vi "SwitchAlias.vi"(0 "reference in":refnum<class "SwitchBase.lvclass">, 1 "Name":string, 2 "Connect":bool, 5 "error in (no error)":errorcluster) -> (14 "reference in":refnum<class "SwitchBase.lvclass">, 19 "error out":errorcluster)   [LabVIEW 2017]
uses:
  SwitchBase.lvclass
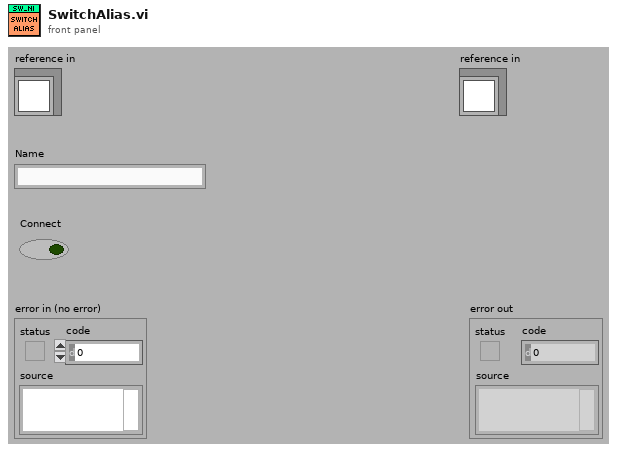
[diagram p1: front panel]
types:
  T1 = typedef "SwitchBase.lvlib/SwitchBase.lvclass/ObjectAttributes.ctl" = cluster{"Config":T2, "History":string[], "channel 1":string, "channel 2":string, "ActiveAlias":string, "AliasState":bool}
  T2 = typedef "SwitchBase.lvlib/SwitchBase.lvclass/Config.ctl" = cluster{"Resource":refnum<k15>, "topology name":T3, "Alias":cluster{"Name":string, "C1,C2":string[][]}[]}
  T3 = typedef "niSwitch Topologies.ctl" = string
  T4 = typedef "SwitchBase.lvlib/SwitchBase.lvclass/ObjectAttributes.ctl" = cluster{"Numeric":dbl}
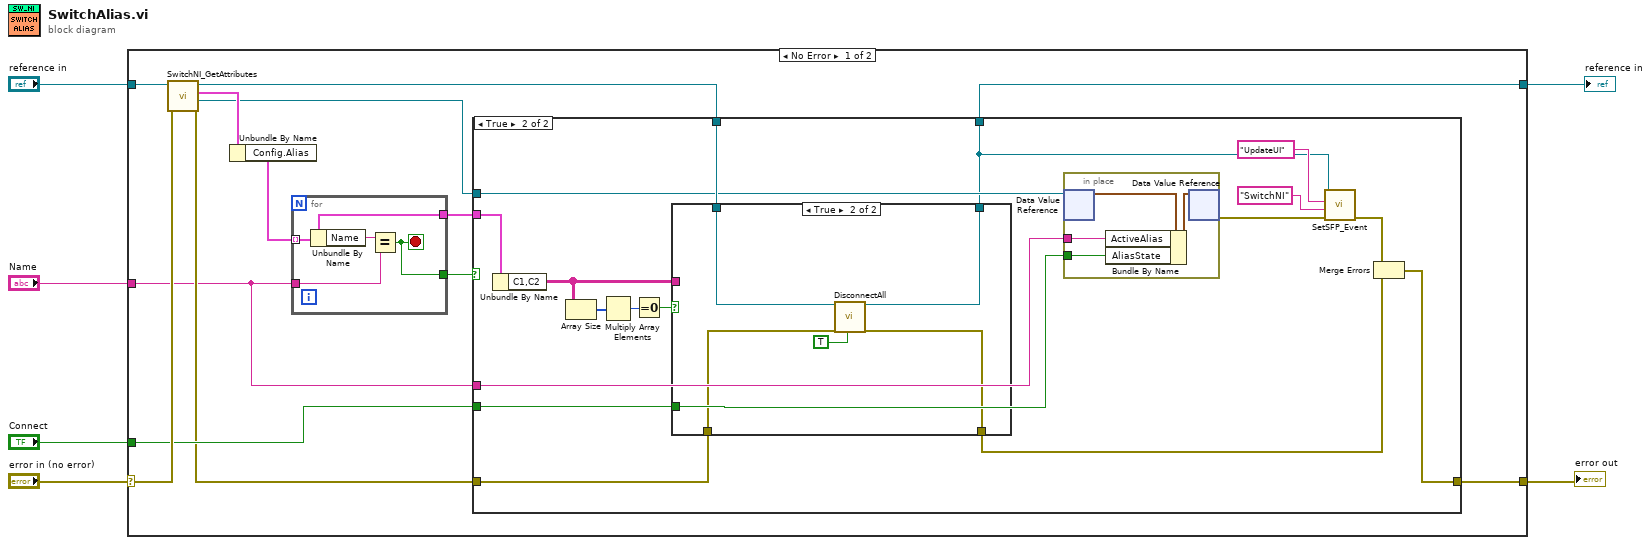
[diagram p0: block diagram]
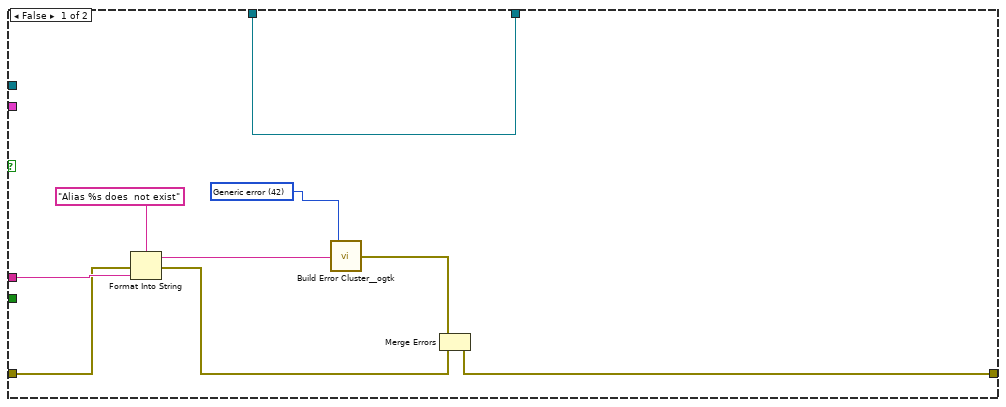
[diagram p2: hidden frame]
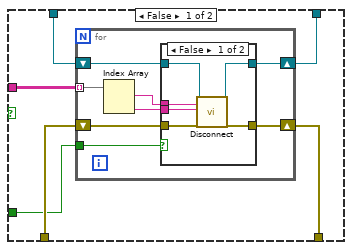
[diagram p3: hidden frame]
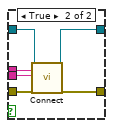
[diagram p4: hidden frame]
diagram:
  n1 = case shown="No Error" "error in (no error)" {
    selector: "error in (no error)" -> [w19 w86]
    tunnel: [w9 w86] -> w5
    tunnel: [w11 w85] -> w3
    tunnel: "reference in" -> [w17 w85]
    tunnel: "Name" -> [w8 _]
    tunnel: "Connect" -> [w13 _]
    frame No Error {
      n2 = call "SwitchNI_GetAttributes.vi"("error in (no error)"=w19, "reference in"=w17) -> ("error out"=w10:errorcluster, "DataRef"=w7:refnum<data-value>, "Data"=w18:T1, "reference out"=w12:refnum<class "SwitchBase.lvclass">)  [unwired: 6 in]
      n3 = Unbundle By Name(w18) -> ("Config.Alias"=w16:cluster{"Name":string, "C1,C2":string[][]}[])
      n4 = for {
        tunnel: w16 -> [w82] mode=indexing
        tunnel: w8 -> [w83]
        tunnel: [w82] -> w14
        tunnel: [w81] -> w15
        stop <- w81 stop-if-true
        n5 = Unbundle By Name(w82) -> ("Name"=w84:string)
        n6 = Equal?(x=w84, y=w83) -> (x = y?=w81:bool)
      }
      n7 = case shown="True" w15 {
        tunnel: w14 -> [_ w43]
        tunnel: w13 -> [_ w40]
        tunnel: w12 -> [w28 w45]
        tunnel: [w28 w29] -> w11
        tunnel: w10 -> [w23 w44]
        tunnel: [w26 w30] -> w9
        tunnel: w8 -> [w24 w41]
        tunnel: w7 -> [_ w42]
        frame False {
          w25 = 42 items=["No error", "Argument error", "Memory is full", "Out of zone", "End of file", "File already open", "Generic file I/O error", "File not found", "File permission error", "Disk is full", "Duplicate path", "Too many files open", "System feature not enabled", "Resource file not found", "Cannot add resource", "Resource not found", "Image not found", "Image memory error", "Pen does not exist", "Config type invalid", "Config token not found", "Config parse error", "Config memory error", "Bad external code format", "Bad external code offset", "External code not present", "Null window", "Destroy window error", "Null menu", "Print aborted", "Bad print record", "Print driver error", "Windows error during printing", "Memory error during printing", "Print dialog error", "Generic print error", "Invalid device refnum", "Device not found", "Device parameter error", "Device unit error", "Cannot open device", "Device call aborted", "Generic error", "Cancelled by user", "Object ID too low", "Object ID too high", "Object not in heap", "Unknown heap", "Unknown object (invalid DefProc)", "Unknown object (DefProc not in table)", "Message out of range", "Invalid (null) method", "Unknown message", "Manager call not supported", "Bad address", "Network operation in progress", "Network operation timed out", "Connection is busy", "Network attribute not supported", "Network error", "Address in use", "System out of memory", "Connection aborted", "Connection refused", "Not connected", "Already connected", "Connection closed", "Initialization error (interapplication manager)", "Bad occurrence", "Wait on unbound occurrence handler", "Occurrence queue overflow", "Datalog type conflict", "Unused", "Unrecognized type (interapplication manager)", "Memory corrupt", "Failed to make temporary DLL", "Old CIN version", "Drag socket not found", "Failed to load drop-object", "Failed to register OLE object", "Failed to release OLE object", "Format specifier type mismatch", "Unknown format specifier", "Too few format specifiers", "Too many format specifiers", "Scan failed", "Newer CIN version", "Error converting to variant", "Runtime menu error", "Password tampered", "Variant attribute not found", "Incompatible variant data type", "Event data is not available", "Event Store is not present", "Occurrence is not found", "Event Queue is not created", "Event info is not available", "Refnum passed is NULL", "Error retrieving Class GUID", "Error retrieving CoClass GUID", "Error retrieving TypeLib GUID.", "Bad built application magic bytes.", "Specific driver is different from the specific driver associated with the Logical Name.", "There is no session opened to the class driver.", "Max Error", "MAX - Error with config objects", "MAX - Error loading configuration", "MAX - Group not supported"]
          n8 = Format Into String(format string="Alias %s does  not exist", error in=w23, w24) -> (resulting string=w20:string, error out=w22:errorcluster)  [unwired: 1 in]
          n9 = call <userlib>:"Build Error Cluster__ogtk.vi"("String to Prepend to source (\"\")"=w20, "code"=w25) -> ("error out"=w27:errorcluster)
          n10 = Merge Errors(w27, w22) -> (w26:errorcluster)
        }
        frame True {
          n11 = Unbundle By Name(w43) -> ("C1,C2"=w39:string[][])
          n12 = Array Size(array=w39) -> (size(s)=w38:i32[])
          n13 = Multiply Array Elements(1:w38) -> (0:w37:i32)
          n14 = Equal To 0?(x=w37) -> (x = 0?=w36:bool)
          n15 = case shown="True" w36 {
            tunnel: w45 -> [w51 w76]
            tunnel: [w50 w75] -> w29
            tunnel: w44 -> [w49 w74]
            tunnel: [w48 w73] -> w32
            tunnel: w40 -> [w47 _]
            tunnel: w39 -> [w46 _]
            frame False {
              n16 = for {
                shift-right: [w58] -> w50
                shift-left: w51 -> [w59]
                shift-right: [w56] -> w48
                shift-left: w49 -> [w57]
                tunnel: w46 -> [w55] mode=indexing
                tunnel: w47 -> [w52]
                n17 = Index Array(array=w55) -> (element #1=w54:string, element #2=w53:string)  [unwired: 2 in]
                n18 = case shown="False" w52 {
                  tunnel: w59 -> [w63 w71]
                  tunnel: [w62 w70] -> w58
                  tunnel: w57 -> [w65 w69]
                  tunnel: [w64 w68] -> w56
                  tunnel: w54 -> [w60 w67]
                  tunnel: w53 -> [w61 w66]
                  frame False {
                    n19 = call-dynamic "Disconnect.vi"("reference in"=w63, "channel 1"=w60, "channel 2"=w61, "error in (no error)"=w65) -> ("reference in"=w62:refnum<class "SwitchBase.lvclass">, "error out"=w64:errorcluster)  [unwired: 14 in]
                  }
                  frame True {
                    n20 = call-dynamic "Connect.vi"("reference in"=w71, "channel 1"=w67, "channel 2"=w66, "error in (no error)"=w69) -> ("reference in"=w70:refnum<class "SwitchBase.lvclass">, "error out"=w68:errorcluster)  [unwired: 14 in]
                  }
                }
              }
            }
            frame True {
              n21 = call-dynamic "DisconnectAll.vi"("reference in"=w76, "error in (no error)"=w74, "WriteHistory"=TRUE) -> ("reference in"=w75:refnum<class "SwitchBase.lvclass">, "error out"=w73:errorcluster)  [unwired: 15 in]
            }
          }
          n22 = in-place {
            in-place-border: w41 -> [w78]
            in-place-border: w40 -> [w77]
            n23 = in-place-dvr #1(w42) -> (w80:T4)  [unwired: 1 out]
            n24 = Bundle By Name(cluster=w80, "ActiveAlias"=w78, "AliasState"=w77) -> (w79:T4)
            n25 = in-place-dvr #1(w79) -> (w33:errorcluster)  [unwired: 1 out]
          }
          n26 = call-dynamic "SetSFP_Event.vi"("error in (no error)"=w33, "Ancestor"="SwitchNI", "msg"="UpdateUI", "reference in"=w29) -> ("error out"=w31:errorcluster)  [unwired: 6 in, 1 out]
          n27 = Merge Errors(w31, w32) -> (w30:errorcluster)
        }
      }
    }
    frame Error {
    }
  }
  "error out" <- w5
  "reference in" <- w3
